vi "Scatter1007.vi"   [LabVIEW 2013]
uses:
  <vilib>/Heliosphere Research LLC/Advanced Plotting Toolkit/api_plotting/ScatterProperties.ctl
  <vilib>/Heliosphere Research LLC/Advanced Plotting Toolkit/properties/Marker.ctl
  <vilib>/Heliosphere Research LLC/Advanced Plotting Toolkit/properties/Marker_Style.ctl
  <vilib>/Heliosphere Research LLC/Advanced Plotting Toolkit/typedefs/PlotColor.ctl
  <vilib>/Heliosphere Research LLC/Advanced Plotting Toolkit/properties/Line.ctl
  <vilib>/Heliosphere Research LLC/Advanced Plotting Toolkit/properties/Line_Style.ctl
  <vilib>/Heliosphere Research LLC/Advanced Plotting Toolkit/properties/Colormap.ctl
  <vilib>/Heliosphere Research LLC/Advanced Plotting Toolkit/properties/Colormap_Map.ctl
  <vilib>/Heliosphere Research LLC/Advanced Plotting Toolkit/properties/Colormap_Scaling.ctl
  <vilib>/Heliosphere Research LLC/Advanced Plotting Toolkit/properties/Display.ctl
  ModeType.ctl
  <vilib>/Heliosphere Research LLC/Advanced Plotting Toolkit/Advanced Plotting Toolkit.lvlib
types:
  T1 = typedef "Advanced Plotting Toolkit.lvlib/PlotColor.ctl" = u32
  T2 = typedef "ModeType.ctl" = enum16{"Normal", "Expected Failure", "Skipped", "Broken"}
  T3 = typedef "Advanced Plotting Toolkit.lvlib/ScatterProperties.ctl" = cluster{"Marker":T4, "Line":T6, "Colormap":T8, "Display":T11}
  T4 = typedef "Advanced Plotting Toolkit.lvlib/Marker.ctl" = cluster{"Style":T5, "Color":T1, "Size":dbl}
  T5 = typedef "Advanced Plotting Toolkit.lvlib/Marker_Style.ctl" = enum16{"Automatic", "Circle", "Square", "Triangle", "Diamond", "Star", "Invisible"}
  T6 = typedef "Advanced Plotting Toolkit.lvlib/Line.ctl" = cluster{"Style":T7, "Color":T1, "Width":sgl}
  T7 = typedef "Advanced Plotting Toolkit.lvlib/Line_Style.ctl" = enum16{"Automatic", "Solid", "Dashed", "Dotted", "Dash-dot", "Invisible"}
  T8 = typedef "Advanced Plotting Toolkit.lvlib/Colormap.ctl" = cluster{"Map":T9, "Value Min":dbl, "Value Max":dbl, "Scaling":T10, "Reverse":bool}
  T9 = typedef "Advanced Plotting Toolkit.lvlib/Colormap_Map.ctl" = enum16{"Automatic", "Rainbow", "Hot and Cold", "White-Black", "White-Blue", "White-Green", "White-Red", "Fire", "Water", "Earth", "Air", "Pastel", "Banded", "Stepped"}
  T10 = typedef "Advanced Plotting Toolkit.lvlib/Colormap_Scaling.ctl" = enum16{"Default"}
  T11 = typedef "Advanced Plotting Toolkit.lvlib/Display.ctl" = cluster{"Alpha":dbl, "Z Order":dbl}
  T12 = typedef "Advanced Plotting Toolkit.lvlib/PlotID.ctl" = i32
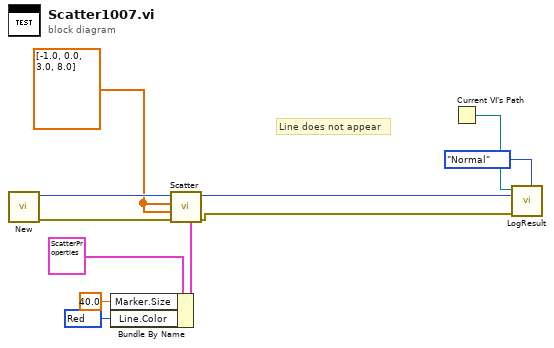
[diagram p0: block diagram]
diagram:
  w1 = T1 16711680 items=["Automatic"=2147483647, "Black"=0, "White"=16777215, "Red"=16711680, "Green"=2263842, "Blue"=255, "Cyan"=65535, "Magenta"=16711935, "Yellow"=16776960] ("Line.Color")
  w6 = dbl[] [-1.0, 0.0, 3.0, 8.0] ("X Data")
  # "Line does not appear"
  n1 = call <vilib>:"New.vi"() -> ("error out"=w9:errorcluster, "Plot ID"=w10:T12)  [unwired: 10 in]
  n2 = Bundle By Name(cluster=T3 {"Marker"={"Style"=enum."Automatic", "Color"=2147483647, "Size"=nan}, "Line"={"Style"=enum."Automatic", "Color"=2147483647, "Width"=nan}, "Colormap"={"Map"=enum."Automatic", "Value Min"=nan, "Value Max"=nan, "Scaling"=enum."Default", "Reverse"=FALSE}, "Display"={"Alpha"=nan, "Z Order"=nan}} ("Scatter Properties"), "Marker.Size"=40.0, "Line.Color"=w1) -> (w4:T3)
  n3 = call <vilib>:"Scatter.vi"("Properties"=w4, "error in (no error)"=w9, "Y Data"=w6, "X Data"=w6, "Plot ID"=w10) -> ("error out"=w7:errorcluster, "Plot ID Out"=w8:T12)  [unwired: 5 in]
  n4 = Current VI's Path() -> (path=w11:path)
  n5 = call "LogResult.vi"("Mode"=ModeType."Normal", "Test Result"=w7, "Test Artifact"=w8, "VI Path"=w11) -> ()  [unwired: 8 in]
